vi "Mutexed Publish Data.vi"(4 "Return Error Transport":refnum<class "ITransport.lvclass">, 6 "Publish Time (Use Current Time)":timestamp, 7 "PublicationPolicy":refnum<class "IPublicationPolicy.lvclass">, 8 "error in (no error)":errorcluster, 9 "Numeric Type":variant, 10 "Datum Name":string, 11 "IModel in":refnum<class "IModel.lvclass">) -> (0 "error out":errorcluster, 3 "IModel out":refnum<class "IModel.lvclass">)   [LabVIEW 2017, in "IModel.lvlib" / "IModel.lvclass"]
uses:
  <vilib>/gpm_packages/@cs/mva-core/Source/IModel/IModel/IModel.lvclass
  C:/Program Files/National Instruments/LabVIEW 2017/vi.lib/gpm_packages/@cs/mva-core/Source/IObserver/IObserver/IObserver.lvclass
  <vilib>/gpm_packages/@cs/mva-core/Source/IMediator/IPublicationPolicy/IPublicationPolicy.lvclass
  <vilib>/gpm_packages/@cs/transport/Source/ITransport/ITransport.lvclass
  <vilib>/gpm_packages/@cs/mva-core/Source/IObserver/IObserver/IObserver.lvclass/IObserver.ctl
  <vilib>/gpm_packages/@cs/mva-core/Source/IModel/IModel/IModel.lvclass/IModel.ctl
  <vilib>/gpm_packages/@cs/mva-core/Source/IMediator/PublishRequest/PublishRequest.lvclass/PublishRequest.ctl
  <vilib>/gpm_packages/@cs/mva-core/Source/IMediator/MutexedPublishRequest/MutexedPublishRequest.lvclass/MutexedPublishRequest.ctl
  <vilib>/gpm_packages/@cs/mva-core/Source/IMediator/IMediator Messages/Publish Msg/Publish Msg.lvclass/Publish Msg.ctl
  <vilib>/gpm_packages/@cs/actor-framework-messages/Source/RoundTripMessage/RoundTripMessage.lvclass/RoundTripMessage.ctl
  <vilib>/ActorFramework/Message Enqueuer/Message Enqueuer.lvclass/Message Enqueuer.ctl
  <vilib>/gpm_packages/@cs/mva-core/Source/IMediator/PublishRequest/Pack Publish Request.vi
  <vilib>/gpm_packages/@cs/actor-framework-messages/Source/RoundTripMessage/Return Round-Trip Message.vi
  <vilib>/ActorFramework/Message Enqueuer/Enqueue.vi
  <vilib>/gpm_packages/@cs/mva-core/Source/IMediator/MutexedPublishRequest/MutexedPublishRequest.lvclass
  C:/Program Files/National Instruments/LabVIEW 2017/vi.lib/gpm_packages/@cs/mva-core/Source/IMediator/PublishRequest/PublishRequest.lvclass
  <vilib>/gpm_packages/@cs/mva-core/Source/IMediator/IMediator Messages/Publish Msg/Publish Msg.lvclass
  C:/Program Files/National Instruments/LabVIEW 2017/vi.lib/gpm_packages/@cs/actor-framework-messages/Source/RoundTripMessage/RoundTripMessage.lvclass
  <vilib>/gpm_packages/@cs/actor-framework-messages/Source/RoundTripMessage/RoundTripMessage.lvclass
  C:/Program Files/National Instruments/LabVIEW 2017/vi.lib/ActorFramework/Message/Message.lvclass
  <vilib>/ActorFramework/Message Priority Queue/Priority Enqueue.vi
  <vilib>/Utility/error.llb/Error Cluster From Error Code.vi
  <vilib>/gpm_packages/@cs/mva-core/Source/IObserver/IObserver/IObserver.lvclass
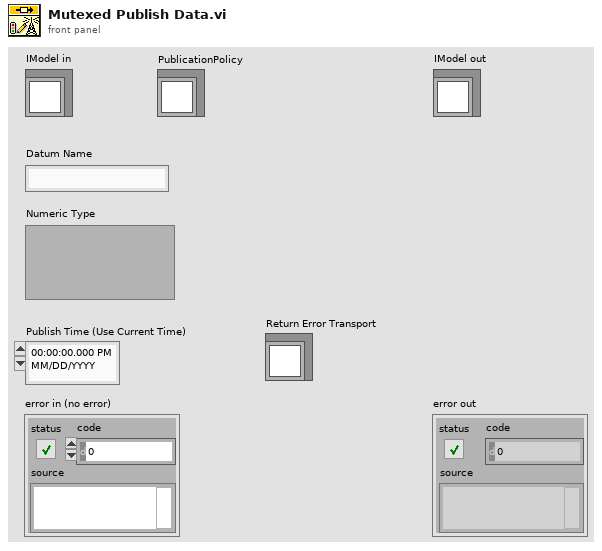
[diagram p1: front panel]
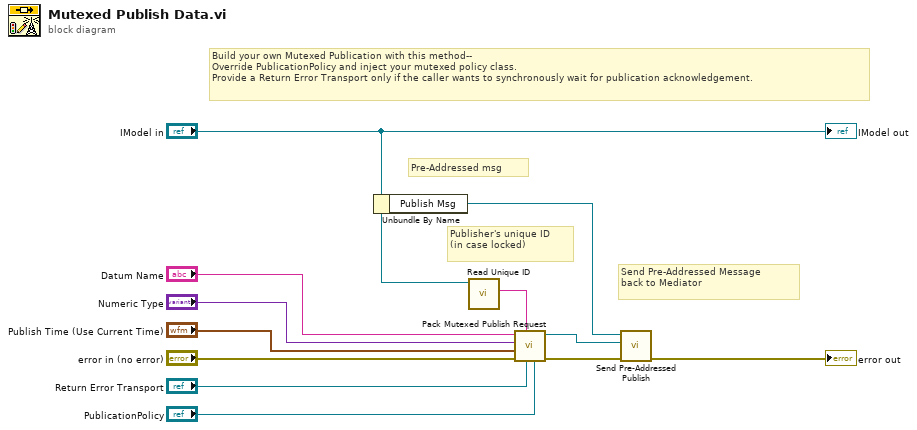
[diagram p0: block diagram]
diagram:
  # "Publisher's unique ID\n(in case locked)"
  # "Pre-Addressed msg"
  # "Send Pre-Addressed Message\nback to Mediator"
  # "Build your own Mutexed Publication with this method--\nOverride PublicationPolicy and inject your mutexed policy class.\nProvide a Return Error Transport only if the caller wants to synchronously wait for publication acknowledgement."
  n1 = Unbundle By Name("IModel in") -> ("Publish Msg"=w6:refnum<class "Publish Msg.lvclass">)
  n2 = call <vilib>:"Read Unique ID.vi"("IObserver In"="IModel in") -> ("Unique ID"=w4:string)  [unwired: 10 in]
  n3 = call <vilib>:"Pack Mutexed Publish Request.vi"("PublicationPolicy"="PublicationPolicy", "Return Error Transport"="Return Error Transport", "Publisher ID"=w4, "error in (no error)"="error in (no error)", "Publish Time (Use Current Time)"="Publish Time (Use Current Time)", "Datum Value or Type"="Numeric Type", "Datum Name"="Datum Name") -> ("error out"=w1:errorcluster, "MutexedPublishRequest Out"=w5:refnum<class "MutexedPublishRequest.lvclass">)  [unwired: 3 in]
  n4 = call <vilib>:"Send Pre-Addressed Publish.vi"("error in (no error)"=w1, "PublishRequest"=w5, "Publish Message"=w6) -> ("error out"=→"error out":errorcluster)  [unwired: 8 in]
  "IModel out" <- "IModel in"
